vi "[NameData] - String Array from Cluster or Enum.vi"(8 "Error":errorcluster, 11 "Enum or\nCluster":variant) -> (0 "Error Out":errorcluster, 3 "Name Array Out":string[](array[string]), 5 "Container name":string)   [LabVIEW 2020]
uses:
  c2264138-84d2-4bed-a5d9-75ac1184d376.vi
  e9b08cd8-247a-46d4-b638-f9fccfba3630.vi
  c2264138-84d2-4bed-a5d9-75ac1184d376.vi/e180abec-803a-4288-9487-3f684c700fb8.vi
  e9b08cd8-247a-46d4-b638-f9fccfba3630.vi/1604689a-0a05-450c-9d40-86f86f38c4fb.vi
  <vilib>/Utility/error.llb/Trim Whitespace.vi
  <vilib>/Utility/Data Type/NI_Data Type.lvlib
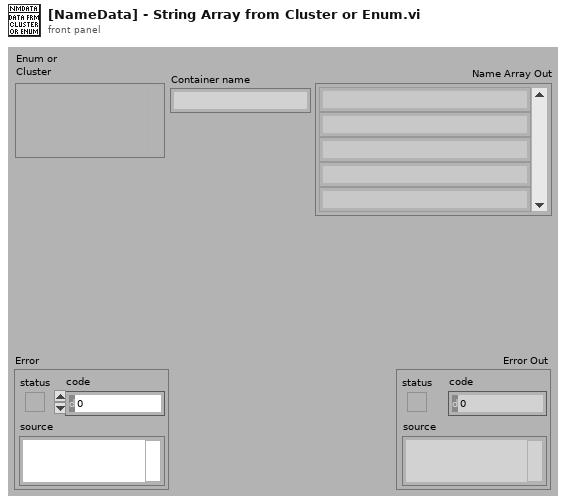
[diagram p1: front panel]
types:
  T1 = typedef "NI_Data Type.lvlib/Data Type.ctl" = enum8{"Invalid Type", "Void", "I8", "I16", "I32", "I64", "U8", "U16", "U32", "U64", "Single Float", "Double Float", "Extended Float", "Single Complex", "Double Complex", "Extended Complex", "Enum U8", "Enum U16", "Enum U32", "Enum U64", "Single Float With Unit", "Double Float With Unit", "Extended Float With Unit", "Single Complex with Unit", "Double Complex with Unit", "Extended Complex with Unit", "Boolean", "String", "Path", "Picture", "Tag", "Array", "Cluster", "Variant", "LV Variant", "Waveform", "Timestamp", "Digital Waveform", "Digital Data", "ExpressData", "Refnum", "External Data", "VI", "Poly VI", "LabVIEW Class Instance", "Fixed Point", "Set Collection", "Map Collection"}
  T2 = typedef "NI_Data Type.lvlib/Type Definition Info.ctl" = cluster{"Name":string, "Timestamp":u32}
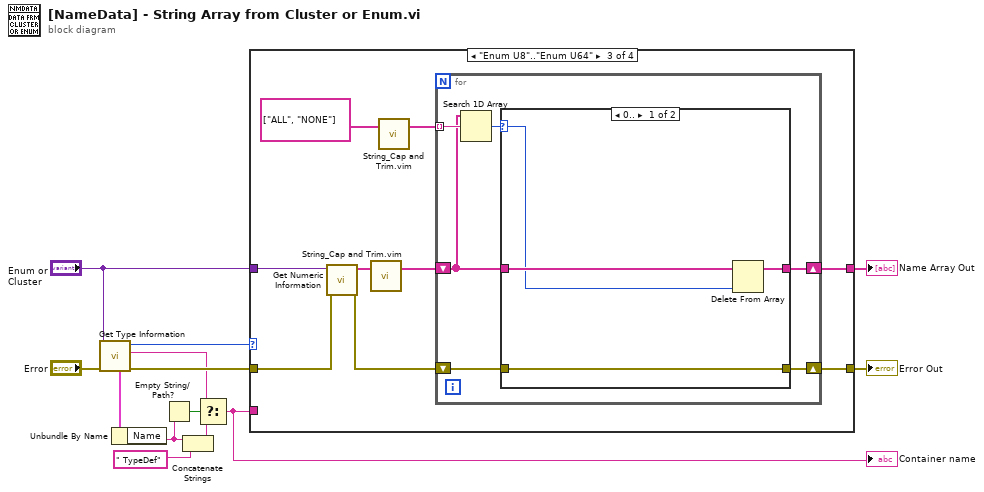
[diagram p0: block diagram]
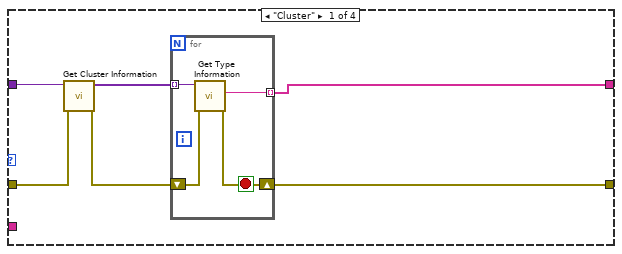
[diagram p2: hidden frame]
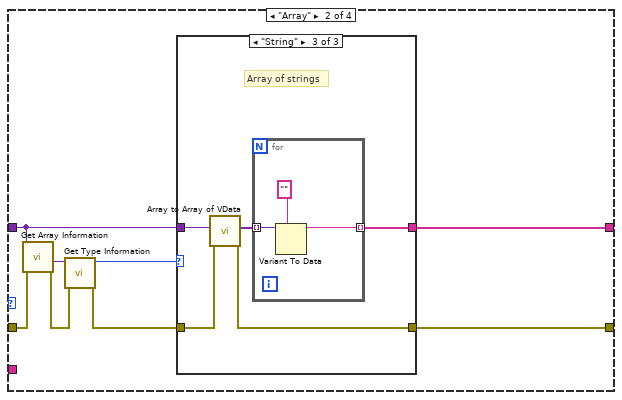
[diagram p3: hidden frame]
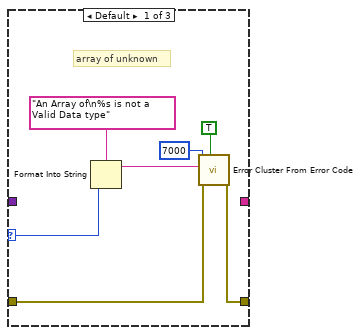
[diagram p4: hidden frame]
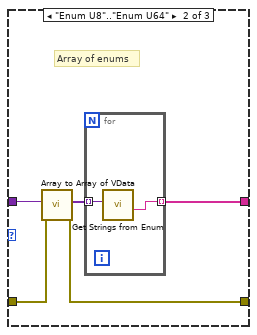
[diagram p5: hidden frame]
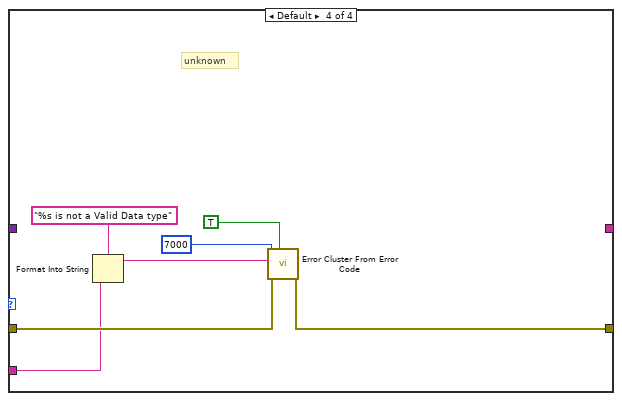
[diagram p7: hidden frame]
diagram:
  n1 = call <vilib>:"Get Type Information.vi"("error in (no error)"="Error", "variant"="Enum or\nCluster") -> ("error out"=w11:errorcluster, "name"=w8:string, "type"=w13:T1, "type definition info"=w9:T2)  [unwired: 5 in, 1 out]
  n2 = Unbundle By Name(w9) -> ("Name"=w5:string)
  n3 = Empty String/Path?(string/path=w5) -> (empty?=w6:bool)
  n4 = Concatenate Strings(w5, " TypeDef" ("string")) -> (w4:string)
  n5 = Select(t=w8, s=w6, f=w4) -> (s? t:f=w7:string)
  "Container name" <- w7
  n6 = case shown="\"Enum U8\"..\"Enum U64\"" w13 {
    tunnel: w11 -> [w18 w30 w61 w77]
    tunnel: "Enum or\nCluster" -> [w19 w31 w62 _]
    tunnel: [w14 w24 w57 _] -> w1
    tunnel: w7 -> [_ _ _ w75]
    tunnel: [w17 w28 w58 w76] -> w2
    frame "Cluster" {
      n7 = call <vilib>:"Get Cluster Information.vi"("error in (no error)"=w18, "variant"=w19) -> ("error out"=w16:errorcluster, "cluster elements"=w15:variant[])  [unwired: 8 in]
      n8 = for {
        shift-right: [w21] -> w17
        shift-left: w16 -> [w22]
        tunnel: w15 -> [w23] mode=indexing
        tunnel: [w20] -> w14 mode=indexing
        stop <- w21 stop-if-true
        n9 = call <vilib>:"Get Type Information.vi"("error in (no error)"=w22, "variant"=w23) -> ("error out"=w21:errorcluster, "name"=w20:string)  [unwired: 5 in, 3 out]
      }
    }
    frame "Array" {
      n10 = call <vilib>:"Get Array Information.vi"("error in (no error)"=w30, "variant"=w31) -> ("error out"=w26:errorcluster, "array element data type"=w29:variant)  [unwired: 6 in, 2 out]
      n11 = call <vilib>:"Get Type Information.vi"("error in (no error)"=w26, "variant"=w29) -> ("error out"=w25:errorcluster, "type"=w27:T1)  [unwired: 5 in, 3 out]
      n12 = case shown="\"String\"" w27 {
        selector: w27 -> [w32 _ _]
        tunnel: w31 -> [_ w43 w50]
        tunnel: [w33 w42 w49] -> w28
        tunnel: w25 -> [w34 w41 w48]
        tunnel: [_ w39 w46] -> w24
        frame Default {
          # "array of unknown"
          n13 = Format Into String(format string="An Array of\n%s is not a Valid Data type" ("error message (\"\")"), w32) -> (resulting string=w36:string)  [unwired: 2 in, 1 out]
          n14 = call <vilib>:"Error Cluster From Error Code.vi"("show call chain? (False)"=TRUE, "error in (no error)"=w34, "error message (\"\")"=w36, "error code (0)"=7000) -> ("error out"=w33:errorcluster)  [unwired: 5 in]
        }
        frame "Enum U8".."Enum U64" {
          # "Array of enums"
          n15 = call "Array to Array of VData.vi"("error in (no error)"=w41, "MultiD Array"=w43) -> ("error out"=w42:errorcluster, "1D Array of Variants"=w40:variant[])  [unwired: 8 in]
          n16 = for {
            tunnel: w40 -> [w45] mode=indexing
            tunnel: [w44] -> w39 mode=indexing
            n17 = call "Get Strings from Enum.vi"("Enum"=w45) -> ("String Value"=w44:string)  [unwired: 7 in, 3 out]
          }
        }
        frame "String" {
          # "Array of strings"
          n18 = call "Array to Array of VData.vi"("error in (no error)"=w48, "MultiD Array"=w50) -> ("error out"=w49:errorcluster, "1D Array of Variants"=w47:variant[])  [unwired: 8 in]
          n19 = for {
            tunnel: w47 -> [w53] mode=indexing
            tunnel: [w51] -> w46 mode=indexing
            n20 = Variant To Data(type="" ("String Value"), Variant=w53) -> (data=w51:string)  [unwired: 1 in, 1 out]
          }
        }
      }
    }
    frame "Enum U8".."Enum U64" {
      n21 = call <vilib>:"Get Numeric Information.vi"("error in (no error)"=w61, "variant"=w62) -> ("error out"=w60:errorcluster, "enum names"=w59:string[])  [unwired: 6 in, 2 out]
      n22 = call "String_Cap and Trim.vim"("String In"=w59) -> ("String Array Out"=w54:string[])  [unwired: 2 in]
      n23 = call "String_Cap and Trim.vim"("String In"=string[] ["ALL", "NONE"]) -> ("String Array Out"=w55:string[])  [unwired: 2 in]
      n24 = for {
        shift-right: [w65] -> w57
        shift-left: w54 -> [w63]
        tunnel: w55 -> [w64] mode=indexing
        shift-right: [w66] -> w58
        shift-left: w60 -> [w67]
        n25 = Search 1D Array(1D array=w63, element=w64) -> (index of element=w68:i32)  [unwired: 1 in]
        n26 = case shown="0.." w68 {
          selector: w68 -> [w70 _]
          tunnel: w67 -> [w72 w74]
          tunnel: [w72 w74] -> w66
          tunnel: w63 -> [w71 w73]
          tunnel: [w69 w73] -> w65
          frame 0.. {
            n27 = Delete From Array(array=w71, index=w70) -> (array with subset deleted=w69:string[])  [unwired: 1 in, 1 out]
          }
          frame ..-1 {
          }
        }
      }
    }
    frame Default {
      # "unknown"
      n28 = Format Into String(format string="%s is not a Valid Data type" ("error message (\"\")"), w75) -> (resulting string=w80:string)  [unwired: 2 in, 1 out]
      n29 = call <vilib>:"Error Cluster From Error Code.vi"("show call chain? (False)"=TRUE, "error in (no error)"=w77, "error message (\"\")"=w80, "error code (0)"=7000) -> ("error out"=w76:errorcluster)  [unwired: 5 in]
    }
  }
  "Name Array Out" <- w1
  "Error Out" <- w2
